vi "PeriodicFilter-Remove Filtered Entry2.vi"(7 "Seconds Since 1Jan1904 2":timestamp, 8 "Settings":T2={"threashold(#/s)"=1.0, "Check Peroid(s)"=1.0}, 9 "State":T1, 11 "Data In":T4 {"LastCheckT" format="%<%.3X>T"}) -> (0 "Removed Info":T3[](array[typedef]), 3 "Data Out":T4 {"LastCheckT" format="%<%.3X>T"})   [LabVIEW 2017, in "Communicable State Machine.lvlib"]
uses:
  Communicable State Machine.lvlib
  Periodic String Filter Data.ctl
  Periodic String Filter Info.ctl
  Periodic String Filter Setting.ctl
  Periodic String Filter State.ctl
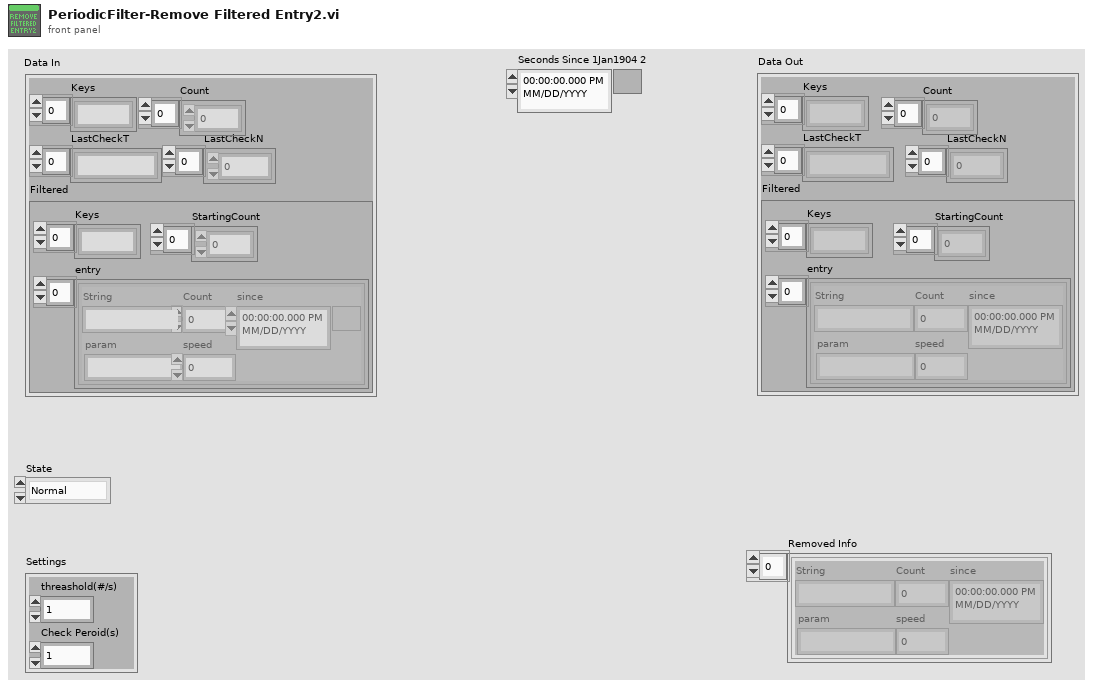
[diagram p1: front panel]
types:
  T1 = typedef "Communicable State Machine.lvlib/Periodic String Filter State.ctl" = enum16{"Normal", "Remove All Filters"}
  T2 = typedef "Communicable State Machine.lvlib/Periodic String Filter Setting.ctl" = cluster{"threashold(#/s)":dbl, "Check Peroid(s)":dbl}
  T3 = typedef "Communicable State Machine.lvlib/Periodic String Filter Info.ctl" = cluster{"String":string, "Count":i64, "since":timestamp, "param":string, "speed":dbl}
  T4 = typedef "Communicable State Machine.lvlib/Periodic String Filter Data.ctl" = cluster{"Keys":string[], "Count":i64[], "LastCheckT":timestamp[], "LastCheckN":i64[], "Filtered":cluster{"Keys":string[], "StartingCount":i64[], "entry":T3[]}}
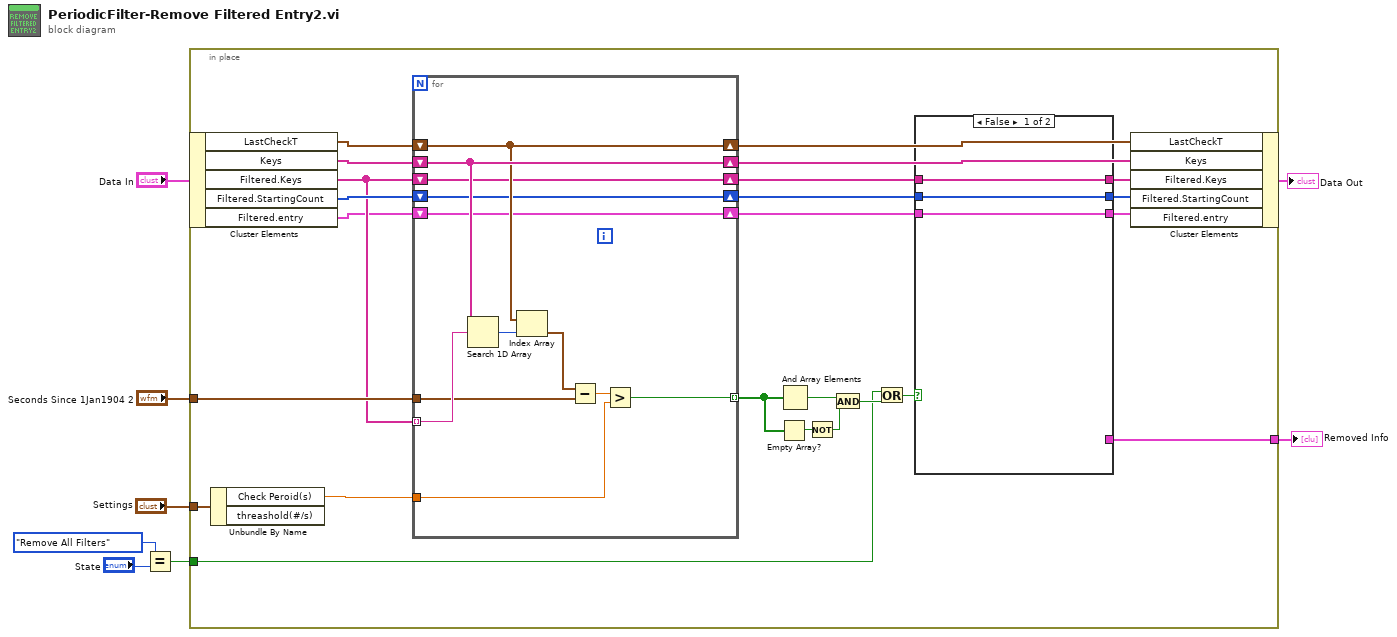
[diagram p0: block diagram]
diagram:
  n1 = Equal?(x=Periodic_String_Filter_State."Remove All Filters", y="State") -> (x = y?=w2:bool)
  n2 = in-place "In Place Element Structure" {
    in-place-border: "Seconds Since 1Jan1904 2" -> [w28]
    in-place-border: "Settings" -> [w27]
    in-place-border: w2 -> [w17]
    in-place-border: [w9] -> w1
    n3 = in-place-cluster #1("Data In") -> ("LastCheckT"=w30:timestamp[], "Keys"=w32:string[], "Filtered.Keys"=w25:string[], "Filtered.StartingCount"=w26:i64[], "Filtered.entry"=w24:T3[])
    n4 = Unbundle By Name(w27) -> ("Check Peroid(s)"=w23:dbl)  [unwired: 1 out]
    n5 = for {
      tunnel: w25 -> [w47] mode=indexing
      shift-right: [w46] -> w31
      shift-left: w32 -> [w46]
      shift-right: [w45] -> w29
      shift-left: w30 -> [w45]
      tunnel: w28 -> [w43]
      shift-right: [w39] -> w12
      shift-left: w26 -> [w39]
      shift-right: [w38] -> w15
      shift-left: w25 -> [w38]
      shift-right: [w40] -> w11
      shift-left: w24 -> [w40]
      tunnel: w23 -> [w41]
      tunnel: [w37] -> w19 mode=indexing
      n6 = Search 1D Array(1D array=w46, element=w47) -> (index of element=w48:i32)  [unwired: 1 in]
      n7 = Index Array(array=w45, index=w48) -> (element=w44:timestamp)
      n8 = Subtract(x=w44, y=w43) -> (x-y=w42:dbl)
      n9 = Greater?(x=w42, y=w41) -> (0:w37:bool)
    }
    n10 = Empty Array?(array=w19) -> (empty?=w21:bool)
    n11 = And Array Elements(Boolean array=w19) -> (logical AND=w22:bool)
    n12 = Not(x=w21) -> (.not. x?=w20:bool)
    n13 = And(x=w22, y=w20) -> (x .and. y?=w18:bool)
    n14 = Or(x=w17, y=w18) -> (x .or. y?=w16:bool)
    n15 = case shown="False" w16 {
      tunnel: w15 -> [w35 _]
      tunnel: [w35 _] -> w14
      tunnel: [w34 _] -> w13
      tunnel: w12 -> [w34 _]
      tunnel: w11 -> [w33 w36]
      tunnel: [w33 _] -> w10
      tunnel: [_ w36] -> w9
      frame False {
      }
      frame True {
      }
    }
    n16 = in-place-cluster #1("LastCheckT"=w29, "Keys"=w31, "Filtered.Keys"=w14, "Filtered.StartingCount"=w13, "Filtered.entry"=w10) -> (→"Data Out":T4)
  }
  "Removed Info" <- w1
